vi "Tosca-Restore Position.vi"(0 "Config":string, 5 "rignum":i32, 11 "error in (no error)":errorcluster) -> (8 "Position":cluster{"Left":i32, "Top":i32}, 15 "error out":errorcluster)   [LabVIEW 2020]
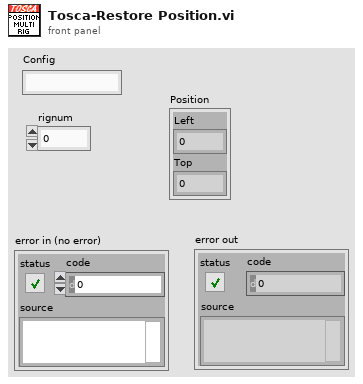
[diagram p1: front panel]
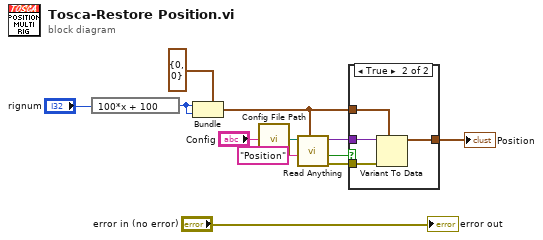
[diagram p0: block diagram]
diagram:
  n1 = expression code="100*x + 100"("rignum") -> (w4:i32)
  n2 = Bundle(cluster=cluster{"Left":i32, "Top":i32} {"Left"=0, "Top"=0} ("Position"), "Left"=w4, "Top"=w4) -> (w1:cluster{"Left":i32, "Top":i32})
  n3 = call "Config File Path.vi"("AppName"="Config") -> ("Default config file name"=w6:path)
  n4 = call "Read Anything.vi"("Type of Anything"=w1, "Section Name (Name of \"Type of Anything\")"="Position" ("Section Name (Name of \"Type of Anything\")"), "Path (dialog)"=w6) -> ("Error Out"=w9:errorcluster, "Found?"=w11:bool, "Anything"=w10:variant)  [unwired: 6 in]
  n5 = case shown="True" w11 {
    tunnel: w9 -> [_ w17]
    tunnel: w10 -> [_ w16]
    tunnel: [w13 w15] -> w5
    tunnel: w1 -> [w13 w14]
    frame False {
    }
    frame True {
      n6 = Variant To Data(error in=w17, type=w14, Variant=w16) -> (data=w15:cluster{"Left":i32, "Top":i32})  [unwired: 1 out]
    }
  }
  "Position" <- w5
  "error out" <- "error in (no error)"
